vi "test_clamp.vi"(0 "Color Plane (Color Plane Extraction 1)":i32(ring)=5 items=["Red", "Green", "Blue", "Hue", "Saturation", "Luminance", "Value", "Intensity"], 1 "ROI Descriptor (Clamp (Rake) 1)":T3={"Global Rectangle"=[68, 155, 773, 255], "Contours"=[{"ID"=enum."External", "Type"=12, "Coordinates"=[68, 155, 773, 255, 0]}]} {"Contours"."Type" items=["No Selection", "Point", "Line", "Rectangle", "Oval", "Polygon", "Freehand Region", "Annulus", "Unused2", "Unused3", "Broken Line", "Freehand Line", "Rotated Rectangle"]}, 2 "Settings (Clamp (Rake) 1)":T2={"Contrast"=40, "Filter width"=4, "Steepness"=2, "Subsampling Ratio"=5, "Show Search Area"=TRUE, "Show Search Lines"=TRUE, "Show Edges Found"=TRUE, "Show Result"=TRUE}) -> (20 "Edge Coordinates (Clamp (Rake) 1)":cluster{"X":sgl, "Y":sgl}[](array[cluster]) {"Y" format="%.2f"; "X" format="%.2f"}, 21 "Edge Coordinates (calibrated) (Clamp (Rake) 1)":cluster{"X":sgl, "Y":sgl}[](array[cluster]) {"Y" format="%.2f"; "X" format="%.2f"}, 22 "Distance (Clamp (Rake) 1)":sgl format="%.2f", 27 "error out":errorcluster)   [LabVIEW 2019]
uses:
  <vilib>/userDefined/High Color/IMAQdx.ctl
  <vilib>/vision/NI_Vision_Development_Module.lvlib
  <vilib>/vision/driver/NI_Vision_Acquisition_Software.lvlib
panel:
  out "error out 2":errorcluster
  in  "millisecond multiple":u32
  in  "stop":bool
  in  "Session In":T1
  out "Image Out":T4(plugin-control)
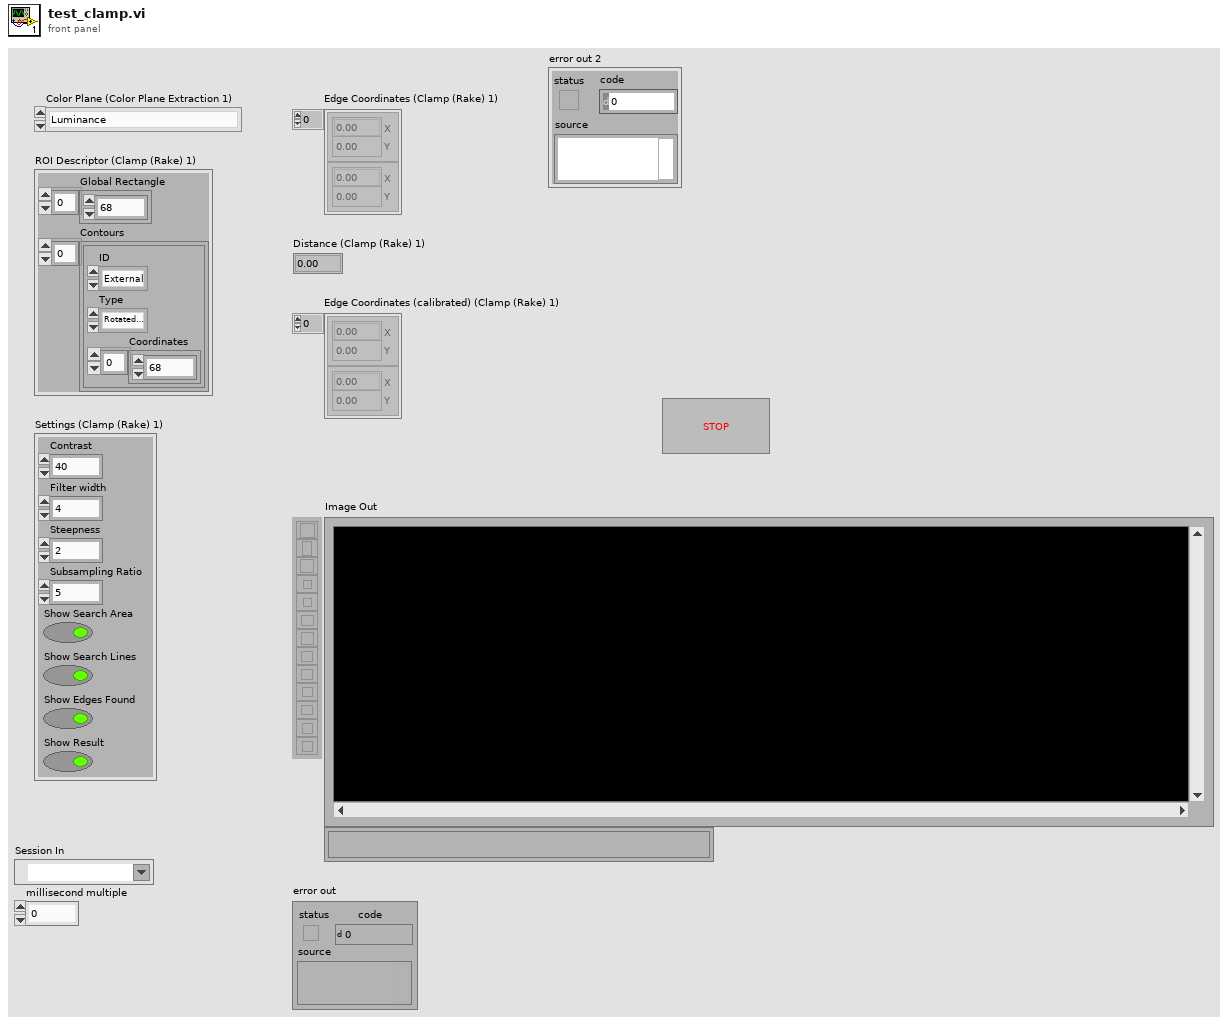
[diagram p1: front panel]
types:
  T1 = typedef "IMAQdx.ctl" = refnum<k21>
  T2 = cluster{"Contrast":i32, "Filter width":i32, "Steepness":i32, "Subsampling Ratio":u32, "Show Search Area":bool, "Show Search Lines":bool, "Show Edges Found":bool, "Show Result":bool}
  T3 = cluster{"Global Rectangle":i32[], "Contours":cluster{"ID":enum32{"External", "Internal"}, "Type":u32, "Coordinates":i32[]}[]}
  T4 = typedef "IMAQ Image.ctl" = refnum<image>
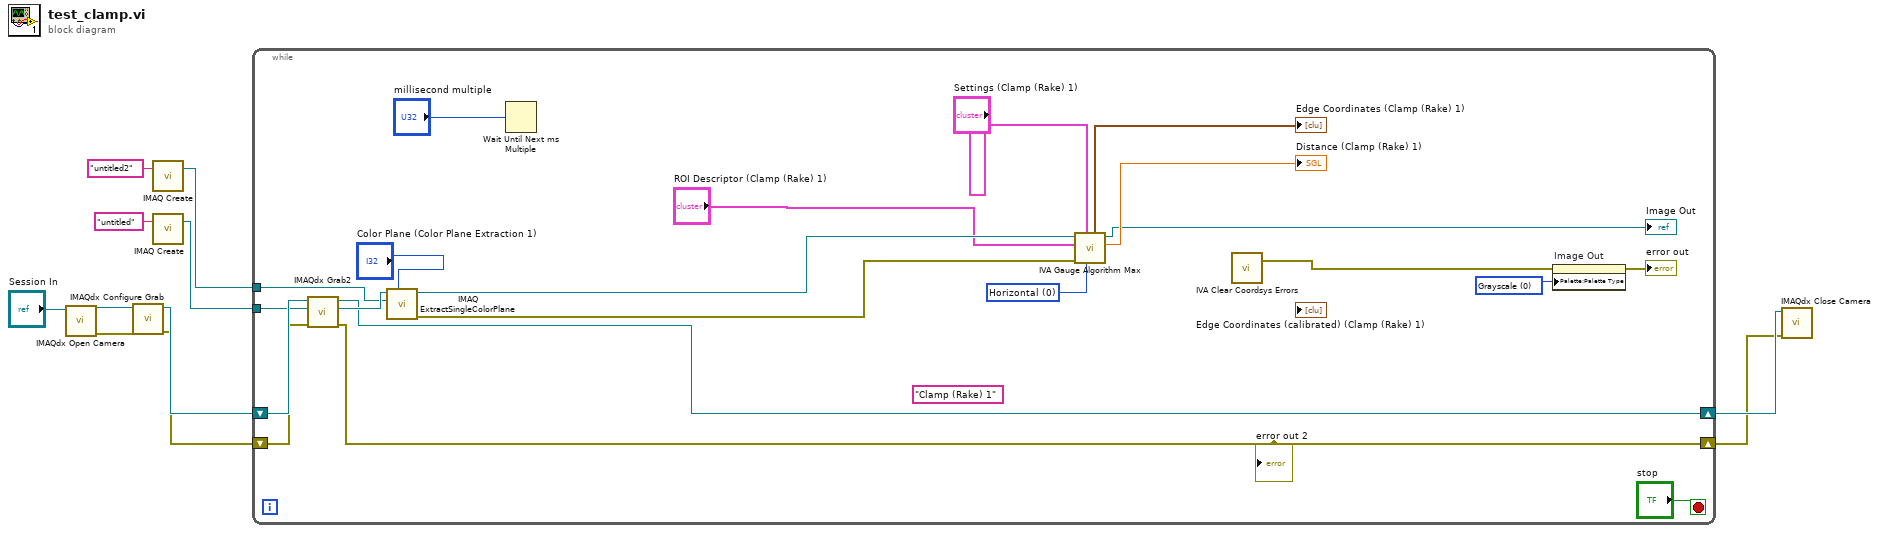
[diagram p0: block diagram]
diagram:
  n1 = call <vilib>:"IMAQdx Open Camera.vi"("Session In"="Session In") -> ("error out"=w11:errorcluster, "Session Out"=w10:T1)  [unwired: 9 in]
  n2 = call <vilib>:"IMAQdx Configure Grab.vi"("error in"=w11, "Session In"=w10) -> ("error out"=w7:errorcluster, "Session Out"=w8:T1)  [unwired: 8 in]
  n3 = call "IMAQ Create"("Image Name"="untitled2") -> ("New Image"=w2:T4)  [unwired: 4 in, 1 out]
  n4 = call "IMAQ Create"("Image Name"="untitled") -> ("New Image"=w6:T4)  [unwired: 4 in, 1 out]
  n5 = while {
    tunnel: w6 -> [w19]
    tunnel: w2 -> [w16]
    shift-right: [w17] -> w3
    shift-left: w8 -> [w21]
    shift-right: [w15] -> w1
    shift-left: w7 -> [w20]
    stop <- "stop" stop-if-true
    w28 = u32 0 items=["Horizontal", "Vertical"] ("Scanning axis (Clamp (Rake) 1)")
    w22 = u32 0 items=["Grayscale", "Binary", "Gradient", "Rainbow", "Temperature", "User Defined", "Binary 16 Bit", "Gradient 16 Bit", "Rainbow 16 Bit", "Temperature 16 Bit", "User Defined 16 Bit"] ("Palette Type")
    (unwired) "Clamp (Rake) 1" ("Step Name")
    n6 = call <vilib>:"IMAQdx Grab2.vi"("error in"=w20, "Image In"=w19, "Session In"=w21) -> ("error out"=w15:errorcluster, "Image Out"=w18:T4, "Session Out"=w17:T1)  [unwired: 5 in, 1 out]
    "error out 2" <- w15
    n7 = call "IMAQ ExtractSingleColorPlane"("Color Plane"="Color Plane (Color Plane Extraction 1)", "Image Dst"=w16, "Image Src"=w18) -> ("error out"=w31:errorcluster, "Image Dst Out"=w30:T4)  [unwired: 1 in, 6 out]
    n8 = Wait Until Next ms Multiple(millisecond multiple="millisecond multiple") -> ()  [unwired: 1 out]
    n9 = call <vilib>:"IVA Gauge Algorithm Max.vi"("Scanning axis"=w28, "Settings"="Settings (Clamp (Rake) 1)", "error in (no error)"=w31, "ROI Descriptor"="ROI Descriptor (Clamp (Rake) 1)", "Image"=w30) -> ("Distance"=→"Distance (Clamp (Rake) 1)":sgl, "Image Out"=→"Image Out":T4, "Points of Contact"=→"Edge Coordinates (Clamp (Rake) 1)":cluster{"X":sgl, "Y":sgl}[])  [unwired: 1 in, 3 out]
    n10 = call <vilib>:"IVA Clear Coordsys Errors.vi"() -> ("error out"=w24:errorcluster)  [unwired: 11 in]
    n11 = property on="Image Out" class="ImageControl"(error in=w24, "Palette:Palette Type"=w22) -> (error out=→"error out":errorcluster)  [unwired: 1 in, 1 out]
  }
  n12 = call <vilib>:"IMAQdx Close Camera.vi"("error in"=w1, "Session In"=w3) -> ()  [unwired: 9 in, 1 out]
